vi "Ejercicio_TablaMultiplicar.vi"() -> ()   [LabVIEW 2020]
panel:
  out "Array":dbl[][](array[numeric])
  in  "Numeric 2":i32
  in  "Numeric":i32
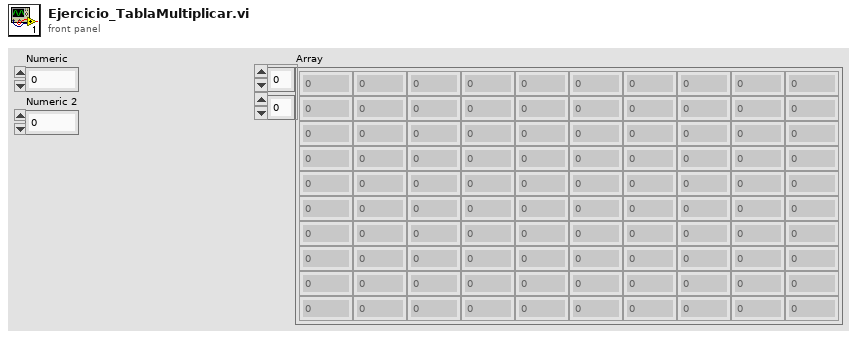
[diagram p1: front panel]
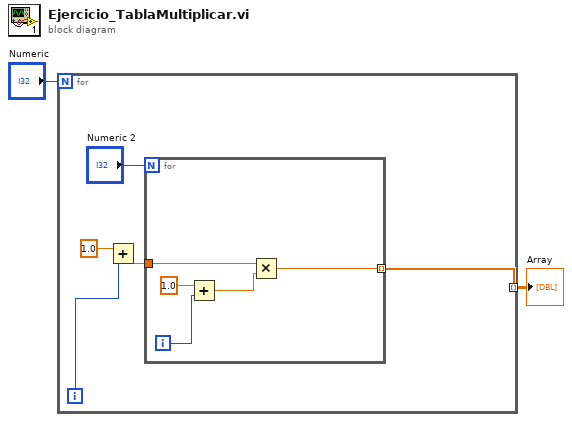
[diagram p0: block diagram]
diagram:
  n1 = for {
    N: "Numeric" -> [_]
    tunnel: [w3] -> w1 mode=indexing
    i -> [w5]
    n2 = Add(x=1.0, y=w5) -> (x+y=w4:dbl)
    n3 = for {
      N: "Numeric 2" -> [_]
      tunnel: w4 -> [w9]
      tunnel: [w8] -> w3 mode=indexing
      i -> [w11]
      n4 = Add(x=1.0, y=w11) -> (x+y=w10:dbl)
      n5 = Multiply(x=w9, y=w10) -> (x*y=w8:dbl)
    }
  }
  "Array" <- w1
